vi "KTable Read Test.vi"() -> ()   [LabVIEW 2015, in "KTable.xctl"]
uses:
  KTable.xctl
  ColumnType.ctl
  ColumnSpec.ctl
panel:
  out "data":cluster{"Val1":string, "Val2":i32, "Val3":T1}[](array[cluster])
  out "Variant":variant
  in  "ColType":T1
  in  "Table Items":string[][](array[string])=[["Shit", "32", "String"]]
  in  "Array":cluster{"Val1":string, "Val2":i32, "Val3":T1}[](array[cluster])
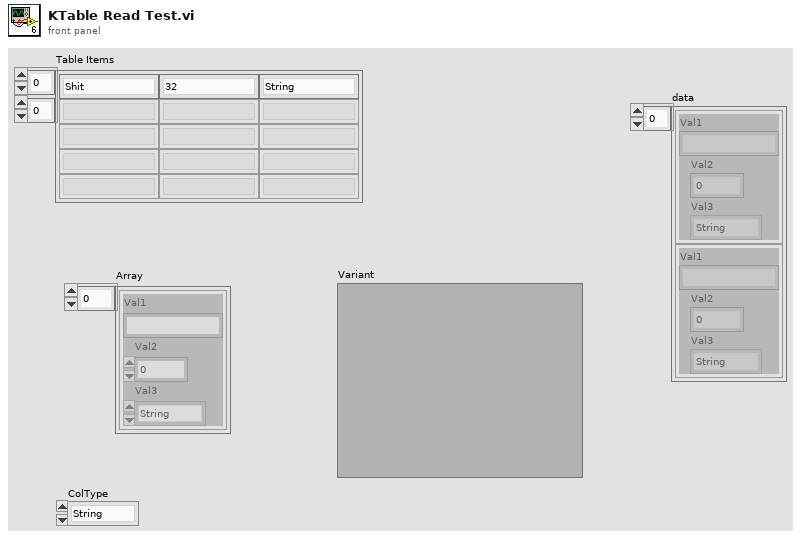
[diagram p1: front panel]
types:
  T1 = typedef "KTable.xctl/ColumnType.ctl" = enum16{"String", "Enum", "Int", "Double", "Boolean", "Ring", "Formula", "Color"}
  T2 = typedef "KTable.xctl/ColumnSpec.ctl" = cluster{"Name":string, "Type":T1, "Width":i32, "Strings":string[], "Position":enum16{"Left", "Center", "Right"}, "locked":bool, "cds":cluster{"Strings":string[]}[][], "Hide NaN":bool}
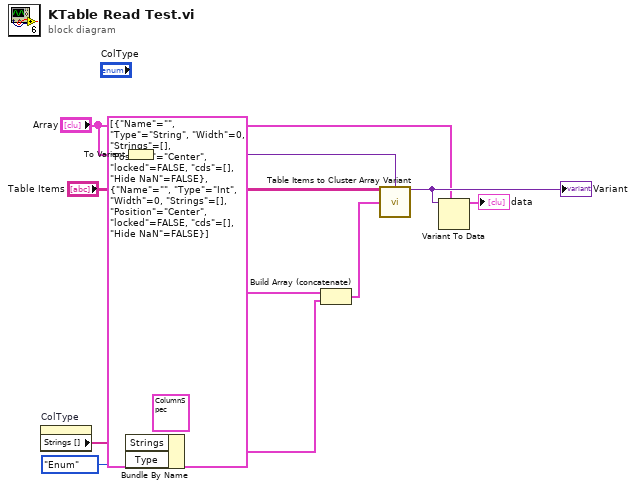
[diagram p0: block diagram]
diagram:
  n1 = property on="ColType" class="Enum (strict)"() -> ("Strings []"=w9:string[])  [unwired: 2 in, 2 out]
  n2 = To Variant(anything="Array") -> (Variant=w6:variant)
  n3 = Bundle By Name(cluster=T2 {"Name"="", "Type"=enum."Enum", "Width"=0, "Strings"=[], "Position"=enum."Center", "locked"=FALSE, "cds"=[], "Hide NaN"=FALSE} ("ColSpec"), "Strings"=w9, "Type"=ColumnType."Enum") -> (w8:T2)
  n4 = Build Array (concatenate)(T2[] [{"Name"="", "Type"=enum."String", "Width"=0, "Strings"=[], "Position"=enum."Center", "locked"=FALSE, "cds"=[], "Hide NaN"=FALSE}, {"Name"="", "Type"=enum."Int", "Width"=0, "Strings"=[], "Position"=enum."Center", "locked"=FALSE, "cds"=[], "Hide NaN"=FALSE}] ("Array"), w8) -> (w7:T2[])
  n5 = call "Table Items to Cluster Array Variant.vi"("Table Items"="Table Items", "Type of Anything"=w6, "Columns"=w7) -> ("Anything"=w3:variant)  [unwired: 11 in, 1 out]
  "Variant" <- w3
  n6 = Variant To Data(type="Array", Variant=w3) -> (data=→"data":cluster{"Val1":string, "Val2":i32, "Val3":T1}[])  [unwired: 1 in, 1 out]
